vi "SetField.vi"(4 "Mode":i32(ring) items=["Persistent", "Driven"], 5 "Approach":i32(ring) items=["Linear", "NoOvershoot", "Oscillate"], 6 "Rate":dbl=100.0, 7 "Field":dbl, 8 "error in (no error)":errorcluster, 9 "Instrument Ref In":refnum<k24>) -> (0 "SetField Error":i32, 2 "error out":errorcluster, 3 "Instrument Ref Out":refnum<k24>)   [LabVIEW 2016]
uses:
  C:/user/patrick/git/PPMS-Monitor-and-Control/lvsrc/drivers/QDInstrument_LabView/QDInstrument.dll
  lvsrc/drivers/QDInstrument_LabView/QDInstrument.dll
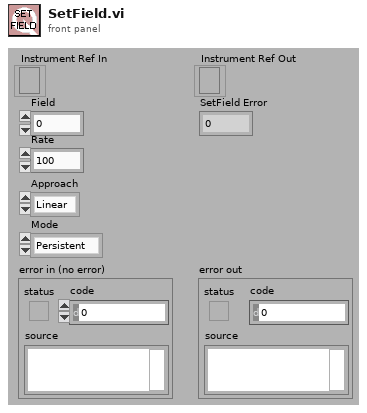
[diagram p1: front panel]
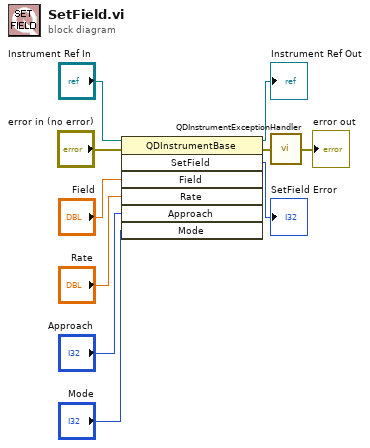
[diagram p0: block diagram]
diagram:
  n1 = invoke class="QDInstrumentBase" method="SetField"(reference="Instrument Ref In", error in="error in (no error)", "Field"="Field", "Rate"="Rate", "Approach"="Approach", "Mode"="Mode") -> (reference out=→"Instrument Ref Out":refnum<k24>, error out=w2:errorcluster, "SetField"=→"SetField Error":i32)  [unwired: 1 in, 4 out]
  n2 = call "QDInstrumentExceptionHandler.vi"("Error in"=w2) -> ("Error out"=→"error out":errorcluster)
